vi "Temperature Monitor.vi"() -> ()   [LabVIEW 2017]
doc: "This VI is the solution to an exercise in the LabVIEW Core 1 course.\n\nIt uses a While Loop and shift registers to average data. No hardware is necessary."
panel:
  in  "Stop Button":bool
  out "Temperature History":cluster{dbl, "Temperature Value":dbl}(graph)
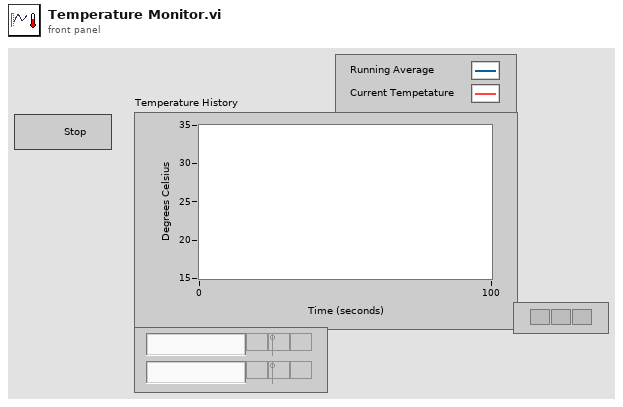
[diagram p1: front panel]
types:
  T1 = enum16{"open", "replace", "create", "open or create", "replace or create", "replace or create with confirmation"}
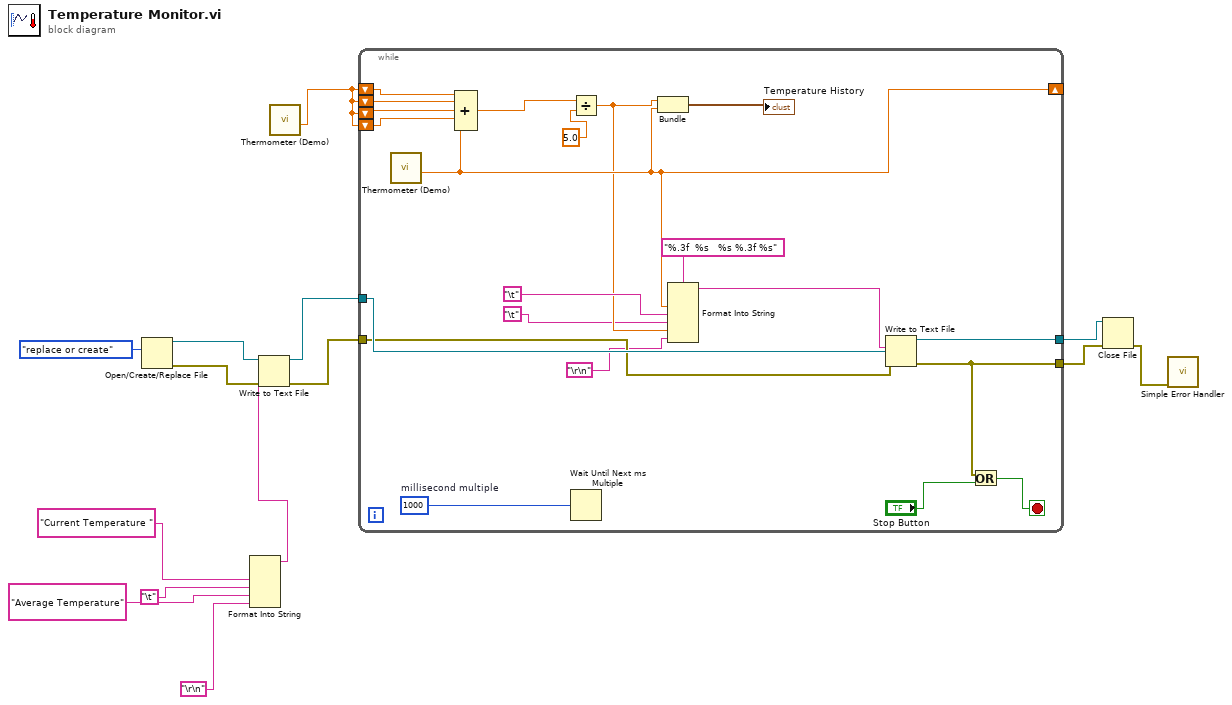
[diagram p0: block diagram]
diagram:
  n1 = Open/Create/Replace File(operation (0:open)=T1."replace or create") -> (refnum out=w9:refnum<file>, error out=w8:errorcluster)  [unwired: 5 in, 1 out]
  n2 = Format Into String("Current Temperature ", "\t", "Average Temperature", "\r\n") -> (resulting string=w4:string)  [unwired: 3 in, 1 out]
  n3 = Write to Text File(file (use dialog)=w9, text=w4, error in=w8) -> (refnum out=w7:refnum<file>, error out=w6:errorcluster)  [unwired: 1 in, 1 out]
  n4 = call "Thermometer (Demo).vi"() -> ("Temperature Value"=w14:dbl)  [unwired: 11 in]
  n5 = while {
    shift-right: [w27] -> _
    shift-left: w14 -> [w34]
    shift-left: w14 -> [w31]
    shift-left: w14 -> [w29]
    shift-left: w14 -> [w30]
    tunnel: w6 -> [w19]
    tunnel: w7 -> [w20]
    tunnel: [w23] -> w12
    tunnel: [w22] -> w11
    stop <- w26 stop-if-true
    w35 = u32 1000  # millisecond multiple
    n6 = call "Thermometer (Demo).vi"() -> ("Temperature Value"=w27:dbl)  [unwired: 11 in]
    n7 = Compound Arithmetic op=ADD(w34, w31, w29, w30, w27) -> (w32:dbl)
    n8 = Divide(x=w32, y=5.0) -> (x/y=w16:dbl)
    n9 = Wait Until Next ms Multiple(millisecond multiple=w35) -> ()  [unwired: 1 out]
    n10 = Bundle(w16, "Temperature Value"=w27) -> (→"Temperature History":cluster{dbl, "Temperature Value":dbl})  [unwired: 1 in]
    n11 = Format Into String(format string="%.3f  %s   %s %.3f %s", w27, "\t", "\t", w16, "\r\n") -> (resulting string=w24:string)  [unwired: 2 in, 1 out]
    n12 = Write to Text File(file (use dialog)=w20, text=w24, error in=w19) -> (refnum out=w23:refnum<file>, error out=w22:errorcluster)  [unwired: 1 in, 1 out]
    n13 = Or(x=w22, y="Stop Button") -> (x .or. y?=w26:bool)
  }
  n14 = Close File(refnum=w12, error in=w11) -> (error out=w10:errorcluster)  [unwired: 1 out]
  n15 = call <vilib>:"Simple Error Handler.vi"("error in (no error)"=w10) -> ()  [unwired: 4 in, 5 out]
